vi "ziExample-HF2-TipProtect.vi"() -> ()   [LabVIEW 2009]
doc: "Control a Zurich instrument device via the LabOne Labview API. \nRequirements: Zurich Instruments HF2.\nThis example controls the Tip Protect settings, which are not avialble in ziControl otherwise. This example is also availalbe in compiled form when ziControl is installed.\n\n© Zurich Instruments AG, www.zhinst.com"
uses:
  <instrlib>/Zurich Instruments LabOne/Public/Configure/ziGetValueString.vi
  <instrlib>/Zurich Instruments LabOne/Public/Configure/ziSetValueDouble.vi
  <instrlib>/Zurich Instruments LabOne/Zurich Instruments LabOne.lvlib
panel:
  in  "stop":bool
  in  "Tab Control":enum32{"TipProtect"}(tab)
  out "pids/%u/tipprotect/active":bool caption="CF"
  out "wasectactive":bool caption="CF"
  in  "clearstatus":bool caption="defaultPhase"
  in  "pids/%u/tipprotect/activetimeconstant":dbl=1.0 caption="TC active (s)" format="%_4p"
  in  "pids/%u/tipprotect/inactivetimeconstant":dbl=0.001 caption="TC inactive (s)" format="%_4p"
  in  "tipprotect_auto_tc":bool caption="LI"
  in  "pids/%u/tipprotect/pll":i32(ring) caption="PLL" items=["1", "2"]
  in  "pids/%u/tipprotect/enable":bool caption="Tip Protect enable"
  in  "pid select":i32(ring) caption="PID" items=["1", "2", "3", "4"]
  out "PID active":bool caption="CF"
  in  "outputdefault":dbl=0.001 caption="Default output value" format="%_4p"
  # "TP active"
  # "PID enabled"
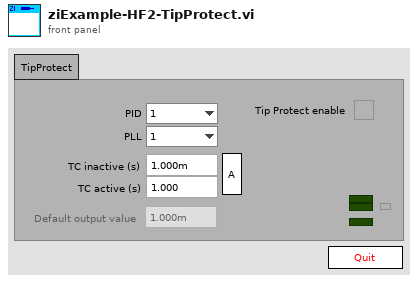
[diagram p1: front panel]
types:
  T1 = typedef "Zurich Instruments LabOne.lvlib/ziTypeHandle.ctl" = cluster{"handleValid":bool, "Conn":u64, "Path Prefix":string, "Handle":u64, "Connected":bool, "Clockbase(s)":dbl}
  T2 = enum32{"invalid app kind", "Development System", "Run Time System", "Student Edition", "Embedded LabVIEW", "Evaluation", "Custom"}
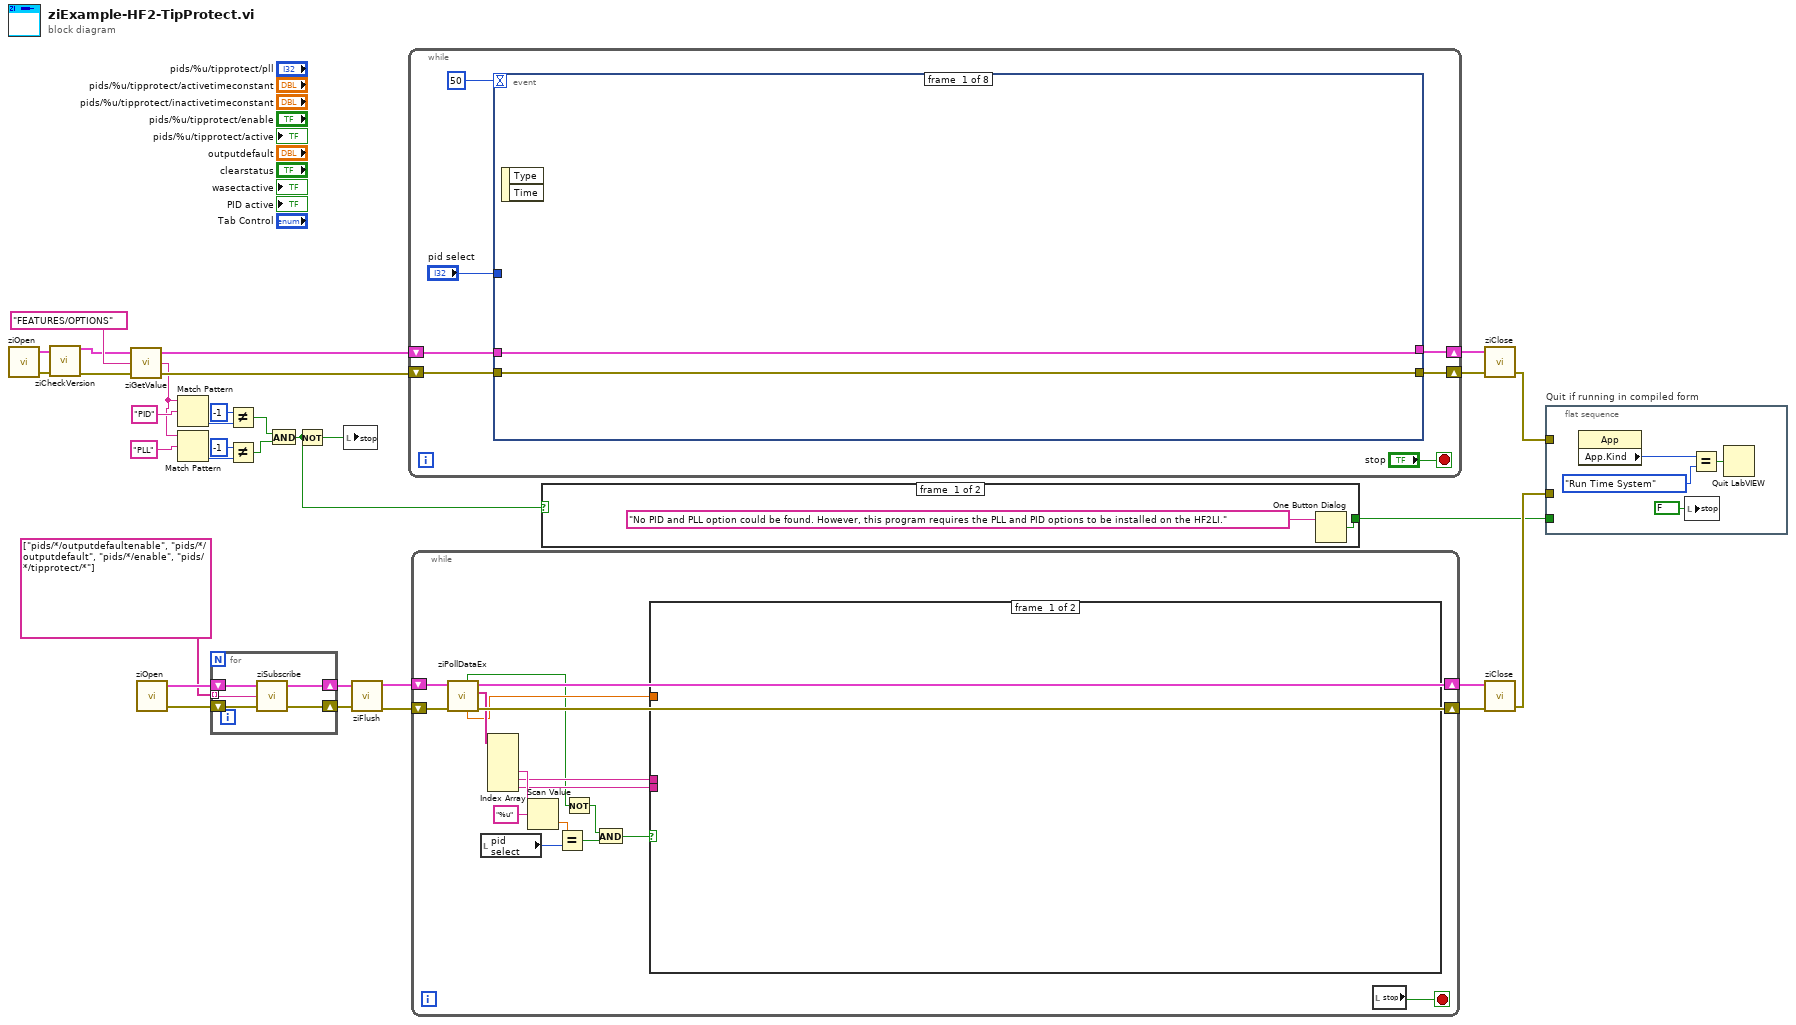
[diagram p0: block diagram]
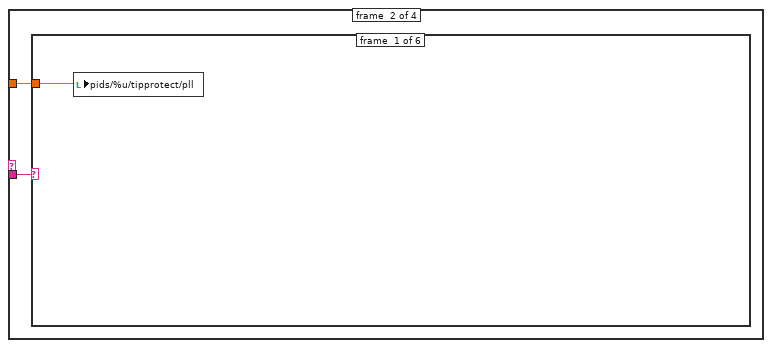
[diagram p4: hidden frame]
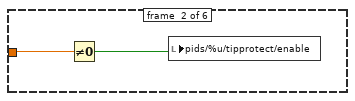
[diagram p5: hidden frame]
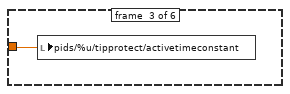
[diagram p6: hidden frame]
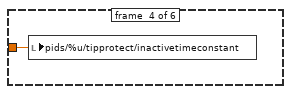
[diagram p7: hidden frame]
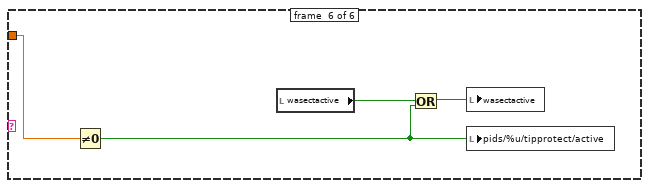
[diagram p9: hidden frame]
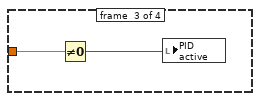
[diagram p10: hidden frame]
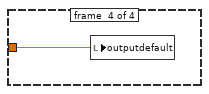
[diagram p11: hidden frame]
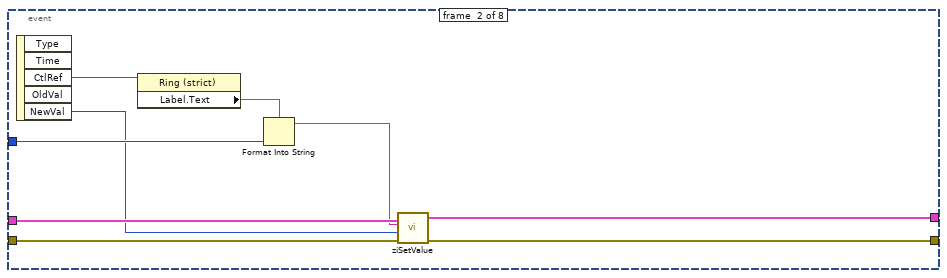
[diagram p12: hidden frame]
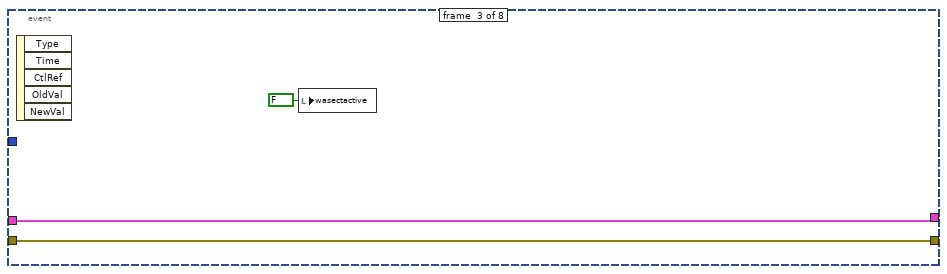
[diagram p13: hidden frame]
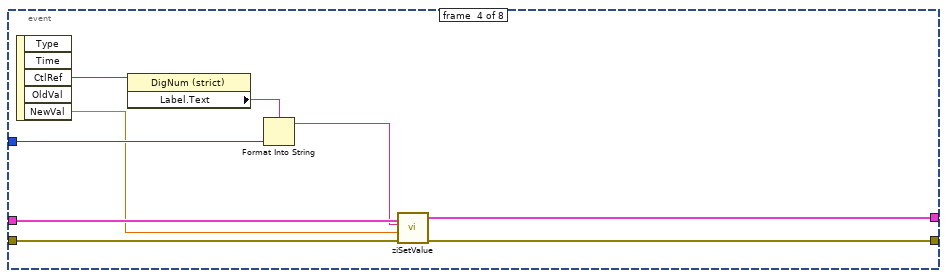
[diagram p14: hidden frame]
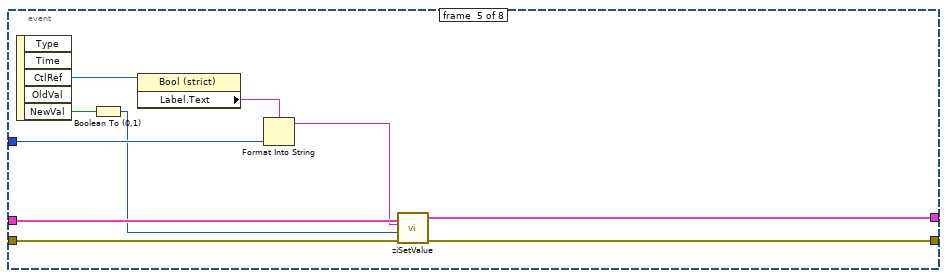
[diagram p15: hidden frame]
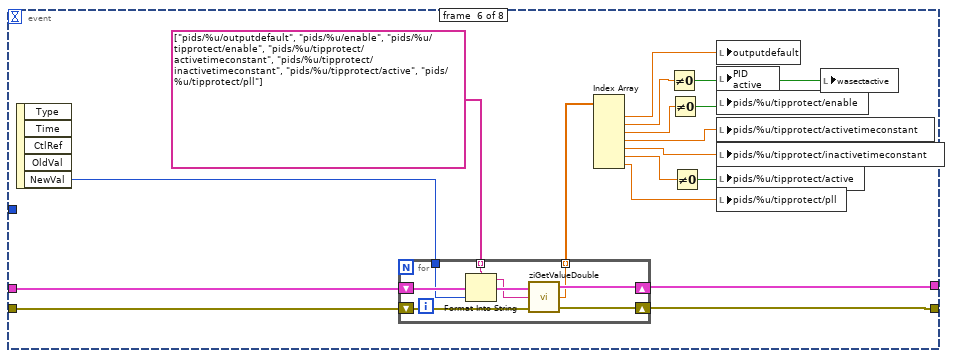
[diagram p16: hidden frame]
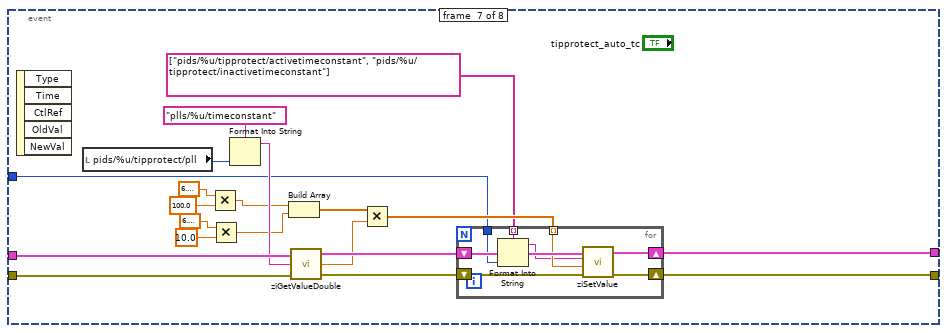
[diagram p17: hidden frame]
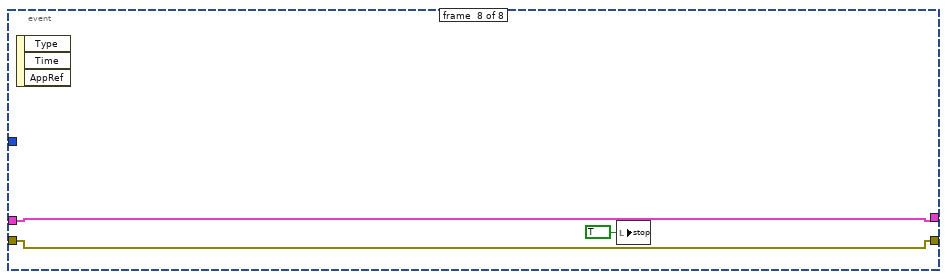
[diagram p18: hidden frame]
diagram:
  n1 = call <instrlib>:"ziOpen.vi"() -> ("Error Out"=w3:errorcluster, "HandleOut"=w4:T1)  [unwired: 4 in, 1 out]
  n2 = call <instrlib>:"ziCheckVersion.vi"("Handle In"=w4, "Error In"=w3) -> ("Handle Out"=w1:T1, "Error Out"=w2:errorcluster)  [unwired: 11 in, 1 out]
  n3 = call-poly <instrlib>:"ziGetValue.vi"("error in"=w2, "Path"="FEATURES/OPTIONS", "Handle In"=w1) -> ("error out"=w18:errorcluster, "Value"=w8:string, "Handle Out"=w19:T1)
  n4 = call <instrlib>:"ziOpen.vi"() -> ("Error Out"=w31:errorcluster, "HandleOut"=w32:T1)  [unwired: 4 in, 1 out]
  n5 = Match Pattern(string=w8, regular expression="PID") -> (offset past match=w14:i32)  [unwired: 4 out]
  n6 = Match Pattern(string=w8, regular expression="PLL") -> (offset past match=w13:i32)  [unwired: 4 out]
  n7 = for {
    tunnel: string[] ["pids/*/outputdefaultenable", "pids/*/outputdefault", "pids/*/enable", "pids/*/tipprotect/*"] -> [w33] mode=indexing
    shift-right: [w35] -> w30
    shift-left: w32 -> [w37]
    shift-right: [w34] -> w29
    shift-left: w31 -> [w36]
    n8 = call <instrlib>:"ziSubscribe.vi"("error in"=w36, "Path ()"=w33, "Handle In"=w37) -> ("error out"=w34:errorcluster, "Handle Out"=w35:T1)  [unwired: 1 in]
  }
  n9 = Not Equal?(x=-1, y=w14) -> (x != y?=w9:bool)
  n10 = Not Equal?(x=-1, y=w13) -> (x != y?=w10:bool)
  n11 = And(x=w9, y=w10) -> (x .and. y?=w6:bool)
  n12 = Not(x=w6) -> (.not. x?=w7:bool)
  n13 = local write "stop"(w7) -> ()
  n14 = call <instrlib>:"ziFlush.vi"("error in"=w29, "Handle In"=w30) -> ("error out"=w27:errorcluster, "Handle Out"=w28:T1)  [unwired: 8 in]
  n15 = while {
    shift-right: [w42] -> w24
    shift-left: w19 -> [w43]
    shift-right: [w41] -> w23
    shift-left: w18 -> [w40]
    stop <- "stop" stop-if-true
    n16 = event shown="[7] Application Instance Close" {
      selector: _ -> [_ _ _ _ _ _ _ _]
      dyn-events: _ -> [_ _ _ _ _ _ _ _]
      timeout: 50 ("TimeOut ms (50)") -> [_ _ _ _ _ _ _ _]
      tunnel: "pid select" -> [_ w53 _ w64 w73 _ w108 _]
      tunnel: w43 -> [w46 w52 w56 w63 w72 w91 w119 w129]
      tunnel: [w46 w51 w56 w62 w71 w90 w115 w129] -> w42
      tunnel: [w45 w50 w55 w61 w70 w88 w114 w128] -> w41
      tunnel: w40 -> [w45 w50 w55 w61 w70 w89 w118 w128]
      event #0 {
        n17 = event-data() -> ()  [unwired: 1 in, 2 out]
      }
      event #1 {
        n18 = event-data() -> ("CtlRef"=w54:refnum<vi>, "NewVal"=w48:i32)  [unwired: 1 in, 3 out]
        n19 = property class="Ring (strict)"(reference=w54) -> ("Label.Text"=w47:string)  [unwired: 1 in, 2 out]
        n20 = Format Into String(format string=w47, w53) -> (resulting string=w49:string)  [unwired: 2 in, 1 out]
        n21 = call-poly <instrlib>:"ziSetValue.vi"("Value"=w48, "Path"=w49, "Handle In"=w52) -> ("Handle Out"=w51:T1)  [unwired: 2 in, 1 out]
      }
      event #2 {
        n22 = event-data() -> ()  [unwired: 1 in, 5 out]
        n23 = local write "wasectactive"(FALSE ("wasectactive")) -> ()
      }
      event #3 {
        n24 = event-data() -> ("CtlRef"=w65:refnum<vi>, "NewVal"=w59:dbl)  [unwired: 1 in, 3 out]
        n25 = property class="DigNum (strict)"(reference=w65) -> ("Label.Text"=w58:string)  [unwired: 1 in, 2 out]
        n26 = Format Into String(format string=w58, w64) -> (resulting string=w60:string)  [unwired: 2 in, 1 out]
        n27 = call-poly <instrlib>:"ziSetValue.vi"("Value"=w59, "Path"=w60, "Handle In"=w63) -> ("Handle Out"=w62:T1)  [unwired: 2 in, 1 out]
      }
      event #4 {
        n28 = event-data() -> ("CtlRef"=w74:refnum<vi>, "NewVal"=w68:bool)  [unwired: 1 in, 3 out]
        n29 = Boolean To (0,1)(Boolean=w68) -> (0, 1=w67:i16)
        n30 = property class="Bool (strict)"(reference=w74) -> ("Label.Text"=w66:string)  [unwired: 1 in, 2 out]
        n31 = Format Into String(format string=w66, w73) -> (resulting string=w69:string)  [unwired: 2 in, 1 out]
        n32 = call-poly <instrlib>:"ziSetValue.vi"("Value"=w67, "Path"=w69, "Handle In"=w72) -> ("Handle Out"=w71:T1)  [unwired: 2 in, 1 out]
      }
      event #5 {
        n33 = event-data() -> ("NewVal"=w76:i32)  [unwired: 1 in, 4 out]
        n34 = for {
          shift-right: [w98] -> w90
          shift-left: w91 -> [w99]
          shift-right: [w96] -> w88
          shift-left: w89 -> [w97]
          tunnel: string[] ["pids/%u/outputdefault", "pids/%u/enable", "pids/%u/tipprotect/enable", "pids/%u/tipprotect/activetimeconstant", "pids/%u/tipprotect/inactivetimeconstant", "pids/%u/tipprotect/active", "pids/%u/tipprotect/pll"] -> [w93] mode=indexing
          tunnel: [w95] -> w86 mode=indexing
          tunnel: w76 -> [w92]
          n35 = Format Into String(format string=w93, w92) -> (resulting string=w94:string)  [unwired: 2 in, 1 out]
          n36 = call <instrlib>:"ziGetValueDouble.vi"("error in"=w97, "Path"=w94, "Handle in"=w99) -> ("error out"=w96:errorcluster, "Value"=w95:dbl, "Handle out"=w98:T1)
        }
        n37 = Index Array(array=w86) -> (element #1=w85:dbl, element #2=w84:dbl, element #3=w82:dbl, element #4=w81:dbl, element #5=w80:dbl, element #6=w78:dbl, element #7=w77:dbl)  [unwired: 7 in]
        n38 = Not Equal To 0?(x=w84) -> (x != 0?=w75:bool)
        n39 = Not Equal To 0?(x=w82) -> (x != 0?=w83:bool)
        n40 = Not Equal To 0?(x=w78) -> (x != 0?=w79:bool)
        n41 = local write "outputdefault"(w85) -> ()
        n42 = local write "PID active"(w75) -> ()
        n43 = local write "pids/%u/tipprotect/enable"(w83) -> ()
        n44 = local write "pids/%u/tipprotect/activetimeconstant"(w81) -> ()
        n45 = local write "pids/%u/tipprotect/inactivetimeconstant"(w80) -> ()
        n46 = local write "pids/%u/tipprotect/active"(w79) -> ()
        n47 = local write "pids/%u/tipprotect/pll"(w77) -> ()
        n48 = local write "wasectactive"(w75) -> ()
      }
      event #6 {
        n49 = event-data() -> ()  [unwired: 1 in, 5 out]
        n50 = local read "pids/%u/tipprotect/pll"() -> (w107:i32)
        n51 = Multiply(x=6.283185307179586, y=100.0 ("x")) -> (x*y=w102:dbl)
        n52 = Multiply(x=6.283185307179586, y=10.0 ("x")) -> (x*y=w101:dbl)
        n53 = Format Into String(format string="plls/%u/timeconstant" ("path"), w107) -> (resulting string=w112:string)  [unwired: 2 in, 1 out]
        n54 = Build Array(w102, w101) -> (w100:dbl[])
        n55 = call <instrlib>:"ziGetValueDouble.vi"("error in"=w118, "Path"=w112, "Handle in"=w119) -> ("error out"=w116:errorcluster, "Value"=w111:dbl, "Handle out"=w117:T1)
        n56 = Multiply(x=w100, y=w111) -> (x*y=w110:dbl[])
        n57 = for {
          tunnel: w110 -> [w123] mode=indexing
          tunnel: string[] ["pids/%u/tipprotect/activetimeconstant", "pids/%u/tipprotect/inactivetimeconstant"] -> [w122] mode=indexing
          shift-right: [w125] -> w115
          shift-left: w117 -> [w127]
          shift-right: [w124] -> w114
          shift-left: w116 -> [w126]
          tunnel: w108 -> [w121]
          n58 = Format Into String(format string=w122, w121) -> (resulting string=w120:string)  [unwired: 2 in, 1 out]
          n59 = call-poly <instrlib>:"ziSetValue.vi"("Error In"=w126, "Value"=w123, "Path"=w120, "Handle In"=w127) -> ("Error Out"=w124:errorcluster, "Handle Out"=w125:T1)  [unwired: 1 in]
        }
      }
      event #7 {
        n60 = event-data() -> ()  [unwired: 1 in, 3 out]
        n61 = local write "stop"(TRUE ("stop")) -> ()
      }
    }
  }
  n62 = while {
    shift-right: [w145] -> w26
    shift-left: w28 -> [w147]
    shift-right: [w144] -> w25
    shift-left: w27 -> [w146]
    stop <- w142 stop-if-true
    n63 = call <instrlib>:"ziPollDataEx.vi"("error in"=w146, "Handle In"=w147) -> ("error out"=w144:errorcluster, "PathArray"=w143:string[], "Handle Out"=w145:T1, "Value Double"=w134:dbl, "Timed Out"=w132:bool)  [unwired: 2 in, 3 out]
    n64 = local read "pid select"() -> (w141:i32)
    n65 = Index Array(array=w143) -> (element #3=w138:string, element #4=w136:string, element #5=w137:string)  [unwired: 5 in, 2 out]
    n66 = Scan Value(string=w138, format string="%u") -> (value=w140:dbl)  [unwired: 1 in, 1 out]
    n67 = Equal?(x=w140, y=w141) -> (x = y?=w135:bool)
    n68 = Not(x=w132) -> (.not. x?=w131:bool)
    n69 = And(x=w131, y=w135) -> (x .and. y?=w133:bool)
    n70 = case shown="True" w133 {
      tunnel: w137 -> [_ w150]
      tunnel: w134 -> [_ w149]
      tunnel: w136 -> [_ w148]
      frame #0 {
      }
      frame #1 {
        n71 = case shown="\"TIPPROTECT\"" w148 {
          tunnel: w150 -> [_ w152 _ _]
          tunnel: w149 -> [_ w151 w163 w164]
          frame #0 {
          }
          frame #1 {
            n72 = case shown="\"INACTIVETIMECONSTANT\"" w152 {
              tunnel: w151 -> [w153 w155 w156 w157 _ w158]
              frame #0 {
                n73 = local write "pids/%u/tipprotect/pll"(w153) -> ()
              }
              frame #1 {
                n74 = Not Equal To 0?(x=w155) -> (x != 0?=w154:bool)
                n75 = local write "pids/%u/tipprotect/enable"(w154) -> ()
              }
              frame #2 {
                n76 = local write "pids/%u/tipprotect/activetimeconstant"(w156) -> ()
              }
              frame #3 {
                n77 = local write "pids/%u/tipprotect/inactivetimeconstant"(w157) -> ()
              }
              frame #4 {
              }
              frame #5 {
                n78 = Not Equal To 0?(x=w158) -> (x != 0?=w159:bool)
                n79 = local read "wasectactive"() -> (w161:bool)
                n80 = Or(x=w161, y=w159) -> (x .or. y?=w160:bool)
                n81 = local write "wasectactive"(w160) -> ()
                n82 = local write "pids/%u/tipprotect/active"(w159) -> ()
              }
            }
          }
          frame #2 {
            n83 = Not Equal To 0?(x=w163) -> (x != 0?=w162:bool)
            n84 = local write "PID active"(w162) -> ()
          }
          frame #3 {
            n85 = local write "outputdefault"(w164) -> ()
          }
        }
      }
    }
    n86 = local read "stop"() -> (w142:bool)
  }
  n87 = case shown="False" w6 {
    tunnel: [w165 _] -> w5
    frame #0 {
      n88 = One Button Dialog(message="No PID and PLL option could be found. However, this program requires the PLL and PID options to be installed on the HF2LI.") -> (true=w165:bool)  [unwired: 1 in]
    }
    frame #1 {
    }
  }
  n89 = call <instrlib>:"ziClose.vi"("Error In"=w23, "Handle In"=w24) -> ("Error Out"=w21:errorcluster)  [unwired: 2 in, 1 out]
  n90 = call <instrlib>:"ziClose.vi"("Error In"=w25, "Handle In"=w26) -> ("Error Out"=w20:errorcluster)  [unwired: 2 in, 1 out]
  n91 = flat-sequence "Quit if running in compiled form" {
    tunnel: w21 -> [_]
    tunnel: w20 -> [_]
    tunnel: w5 -> [_]
    frame #0 {
      n92 = property class="App"() -> ("App.Kind"=w170:T2)  [unwired: 2 in, 2 out]
      n93 = local write "stop"(FALSE ("stop")) -> ()
      n94 = Equal?(x=w170, y=T2."Run Time System" ("Application:Kind")) -> (x = y?=w168:bool)
      n95 = Quit LabVIEW(quit? (T)=w168) -> ()
    }
  }
